vi "Send Items Double Click.vi"(4 "Row":i32, 5 "PlatMods":T1, 6 "Mods":cluster{"Double Click":bool, "Menu Key":bool}, 7 "Message Priority (Normal)":T3=enum."Normal", 8 "error in (no error)":errorcluster, 9 "Button":u16, 10 "Coords":T2, 11 "Message Enqueuer":refnum<class "Message Enqueuer.lvclass">) -> (0 "error out":errorcluster, 3 "Message Enqueuer out":refnum<class "Message Enqueuer.lvclass">)   [LabVIEW 2016, in "Items Double Click Msg.lvclass"]
doc: "This VI sends the message to an actor."
uses:
  Items Double Click Msg.lvclass
  <vilib>/ActorFramework/Message Enqueuer/Message Enqueuer.lvclass
  <vilib>/ActorFramework/Message Enqueuer/Message Priority.ctl
  <vilib>/Utility/miscctls.llb/LVPoint32TypeDef.ctl
  D:/Program Files/National Instruments/LabVIEW 2016/vi.lib/ActorFramework/Message/Message.lvclass
  Items Double Click Msg.lvclass/Items Double Click Msg.ctl
  <vilib>/ActorFramework/Message Enqueuer/Message Enqueuer.lvclass/Message Enqueuer.ctl
  <vilib>/ActorFramework/Message Priority Queue/Priority Enqueue.vi
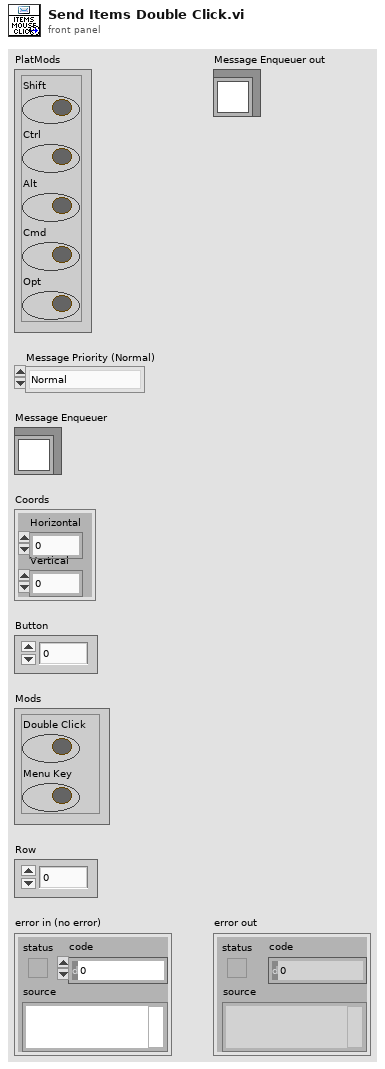
[diagram p1: front panel]
types:
  T1 = cluster{"Shift":bool, "Ctrl":bool, "Alt":bool, "Cmd":bool, "Opt":bool}
  T2 = typedef "LVPoint32TypeDef.ctl" = cluster{"Horizontal":i32, "Vertical":i32}
  T3 = typedef "Actor Framework.lvlib/Message Enqueuer.lvclass/Message Priority.ctl" = enum16{"Low", "Normal", "High"}
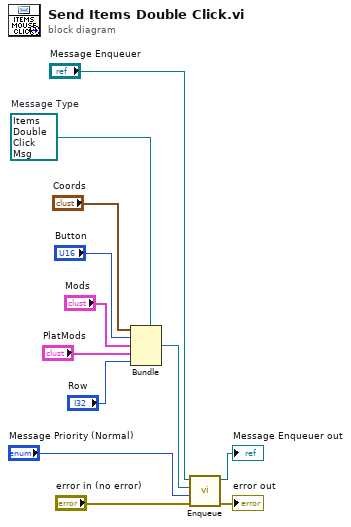
[diagram p0: block diagram]
diagram:
  w9 = refnum<class "Items Double Click Msg.lvclass"> refnum  # Message Type
  n1 = Bundle(cluster=w9, "Coords", "Button", "Mods", "PlatMods", "Row") -> (w8:refnum<class "Items Double Click Msg.lvclass">)
  n2 = call <vilib>:"Enqueue.vi"("error in (no error)"="error in (no error)", "Message Priority (Normal)"="Message Priority (Normal)", "Message"=w8, "Message Enqueuer in"="Message Enqueuer") -> ("error out"=→"error out":errorcluster, "Message Enqueuer out"=→"Message Enqueuer out":refnum<class "Message Enqueuer.lvclass">)  [unwired: 6 in]
